vi "STA - Wave V5 Host_Wait_V2.2.vi"() -> ()   [LabVIEW 2015]
doc: "The continuous acquisition mode tells the FPGA to acquire points indefinitely until a stop command is issued or until an error is encountered (FIFO overflow, module underflow, and so on). \n\nIn this acquisition mode, explicitly call the appropriate rwfm_ConfigTiming VI and set the host application's data buffer to be many times larger than the read size. The examples use a 10X size by default. If the host application's data buffer fills, then the FPGA experiences a FIFO overflow causing the acquisition to stop."
uses:
  <vilib>/LabVIEW Targets/FPGA/cRIO/shared/nicrio_ModuleControls/nicrio_cRIO-9234_ConfigModeRing.ctl
  <vilib>/Platform/TimedLoop/XDataNode/timing_clust.ctl
  <vilib>/Platform/TimedLoop/XDataNode/nitl_modes.ctl
  <vilib>/Platform/TimedLoop/XDataNode/wakeup.ctl
  <vilib>/FPGAPlugInAG/cRIO-9112/niLvFpga_Open_cRIO-9112.vi
  <vilib>/rvi/interface/common/dynamic/niFpgaDynamicAddResources.vi
  <vilib>/Utility/error.llb/Error Cluster From Error Code.vi
  <vilib>/RVI Host/nirviSupport.llb/nirviErrorClusterFromErrorCode.vi
  <vilib>/rvi/errors/niLvFpgaAdjustHostInterfaceError.vi
  <vilib>/FPGAPlugInAG/Dynamic/niLvFpga_Close_Dynamic.vi
  <vilib>/rvi/interface/nirviOpenFPGA/nirviOpenFPGA.xnode
  FPGA Bitfiles/STA-WaveformV5_FPGATarget2_[FPGA]DeltaSigMa_sLRIAVfzKK0.lvbitx
  FPGA/[FPGA] DeltaSig Main V5.vi
  <vilib>/rvi/interface/nirviMethod/nirviMethod.xnode
  <vilib>/rvi/interface/nirviCloseFPGA/nirviCloseFPGA.xnode
  <vilib>/Platform/TimedLoop/XDataNode/XDataNode.xnode
  <vilib>/NI/cRIO Wfm/cRIO Wfm.lvlib
  <vilib>/rvi/interface/nirviMethod/StockFPGA_InlinedMethodWaitForSingleIRQ.vi
  <vilib>/FPGAPlugInAG/Dynamic/niLvFpga_WaitOnIrq_Dynamic.vi
  C:/Program Files (x86)/National Instruments/LabVIEW 2015/ProjectTemplates/Source/cRIOWfm/FPGA/[FPGA] SAR Acq Main.vi
  D/Documents/LabVIEW Data/STA - Waveform V0/FPGA Bitfiles/SARAcqMain_9074.lvbitx
  <vilib>/Platform/TimedLoop/XDataNode/XDNodeRunTimeDep.lvlib
panel:
  out "x > y?":bool
  out "error TDMS":errorcluster
  in  "base path":path=path "u:/"
  out "file path":path
  out "Size Waveform":i32
  out "size(s) 2":i32[](array[numeric])
  out "Y":sgl[][](array[numeric])
  in  "appended array 2":sgl[](array[numeric])
  out "appended array":sgl[](array[numeric])
  out "size(s)":i32[](array[numeric])
  out "i RT FIFO Read":i32
  out "Element 2":u32
  out "Element 1":u32
  out "transposed array":sgl[][](array[numeric])
  out "error out 2":errorcluster
  out "error out":errorcluster
  out "error fifo out":errorcluster
  out "Waveform Graph 2":sgl[][](graph)
  in  "Array":waveform(sgl)[](array[waveform])
  out "Waveform Graph":waveform(sgl)[](graph)
  out "Buffer Backlog":dbl caption="RT Buffer Backlog [%]" format="%#.2g"
  in  "Stop":bool
  in  "Amplitude":dbl(slide)=5.0 scale=0.0..10.0
  out "Time Measure":dbl
  out "data rate (S/s)":u32
  out "Channel Config":T2(array[cluster]) {"Input Configuration" items=["AC Coupled", "DC Coupled", "IEPE AC Coupled"]}
  in  "Samples per Read":i32=900
  # "Sampling Info"
  # "Channel Info"
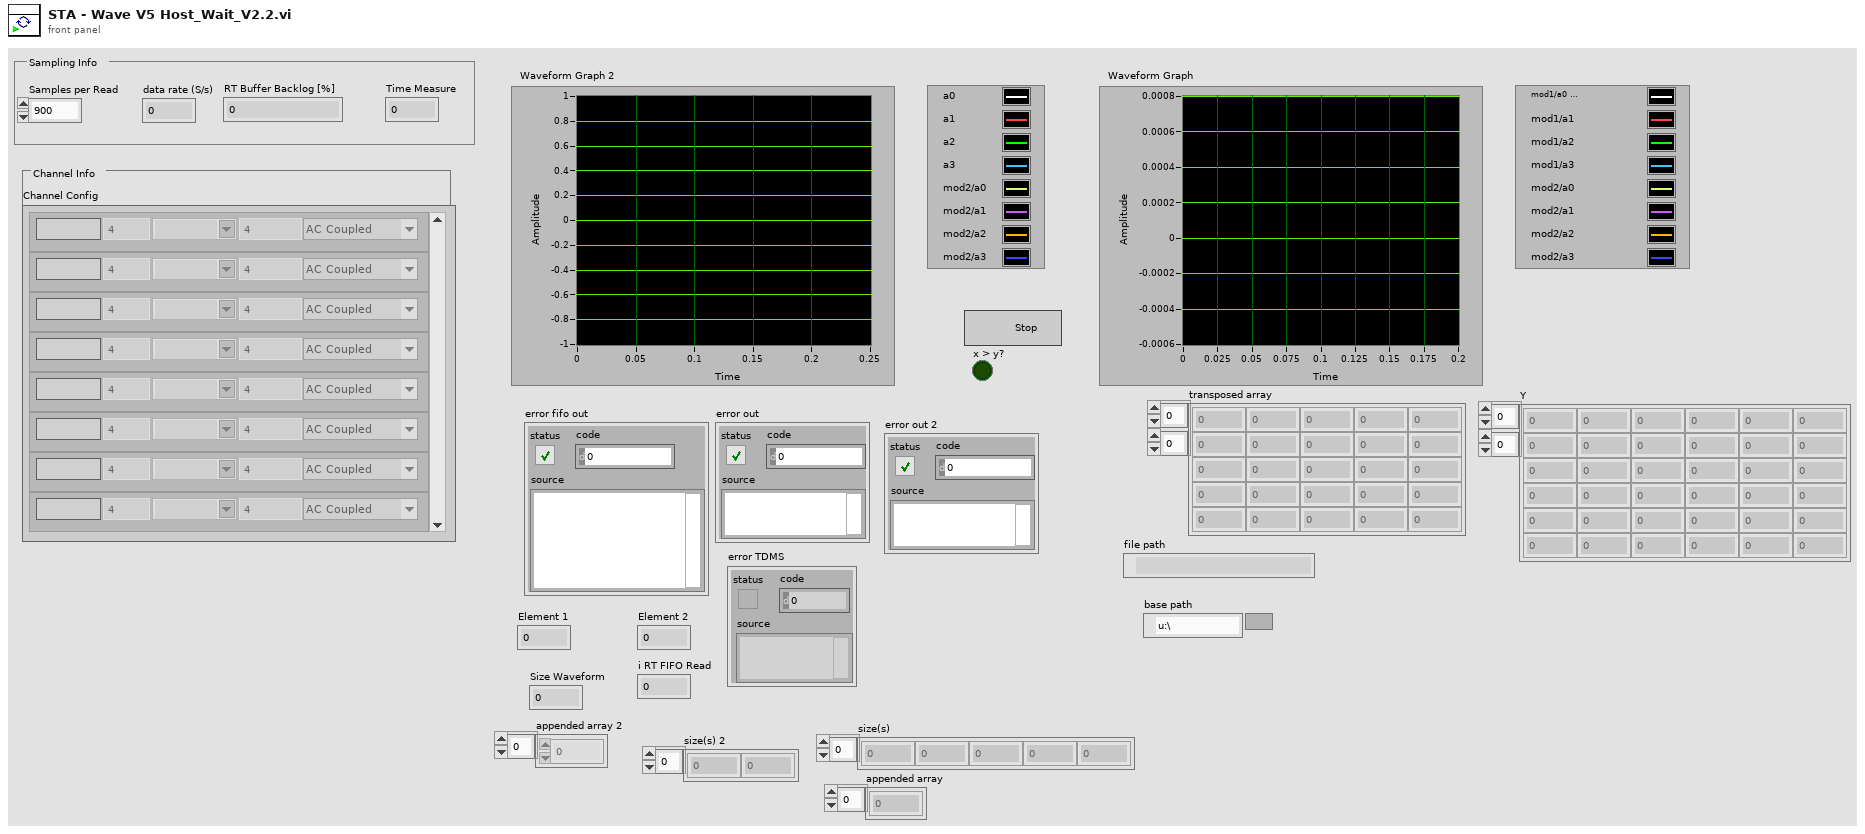
[diagram p1: front panel]
types:
  T1 = typedef "nicrio_cRIO-9234_ConfigModeRing.ctl" = u8
  T2 = cluster{"Channel Name":string, "Sensitivity mV_EU":dbl, "EU":string, "Input Configuration":T1, "dB Ref EU":dbl}[]
  T3 = enum16{"open", "open or create", "create or replace", "create", "open (read-only)"}
  T4 = typedef "XDNodeRunTimeDep.lvlib/timing_clust.ctl" = cluster{"Expected End [f-1]":u64, "Actual End [f-1]":u64, "Finished Late? [f-1]":bool, "Expected End [i-1]":u64, "Actual End [i-1]":u64, "Finished Late? [i-1]":bool, "Expected Start [i]":u64, "Actual Start [i]":u64, "Expected Start [f]":u64, "Actual Start [f]":u64, "Source Name":string, "Structure Name":string, "Period":i64, "Deadline":i64, "Offset":i64, "Start":i64, "Priority":i32, "Timeout":i32, "Mode":T5, "Wakeup Reason":T6, "Error":errorcluster, "Source Type":string, "Secondary Source Type":string, "Global End Time":u64, "Global Start Time":u64, "Frame Duration":u64, "Iteration Duration":u64, "Assigned CPU":i32, "I/O Scan Engine Mode":u32}
  T5 = typedef "XDNodeRunTimeDep.lvlib/nitl_modes.ctl" = enum32{"No Change", "Process missed periods, maintain original phase", "Discard missed periods, maintain original phase", "Process missed periods, ignore original phase", "Discard missed periods, ignore original phase"}
  T6 = typedef "XDNodeRunTimeDep.lvlib/wakeup.ctl" = enum32{"Normal", "Aborted", "Asynchronous wakeup", "Timing source error", "Timed loop error", "Timeout"}
  T7 = typedef "Acquisition and Logging Configuration_Waveform.ctl" = cluster{"Samples per Read":i32, "Number of Reads to Save":i32, "Data File Name":string, "TDMS Properties":T8[], "Number of Channels":i32, "Trigger - RMS Value":dbl, "Trigger - Channel":i32, "Trigger - Time (Minute)":i32, "Channel Config":cluster{"Channel Name":string, "Sensitivity mV_EU":dbl, "EU":string, "Input Configuration":T1, "dB Ref EU":dbl}[], "data rate (S/s)":u32, "Time Measure":dbl}
  T8 = typedef "TDMS Properties.ctl" = cluster{"Name":string, "Value":string}
  T9 = typedef "cRIO Wfm.lvlib/SamplingInfo.ctl" = cluster{"Number of Channels":i32, "Actual Samp Rate":dbl, "Chan Name Array":string[], "EU Chan Array":string[], "dB Ref Chan Array":dbl[]}
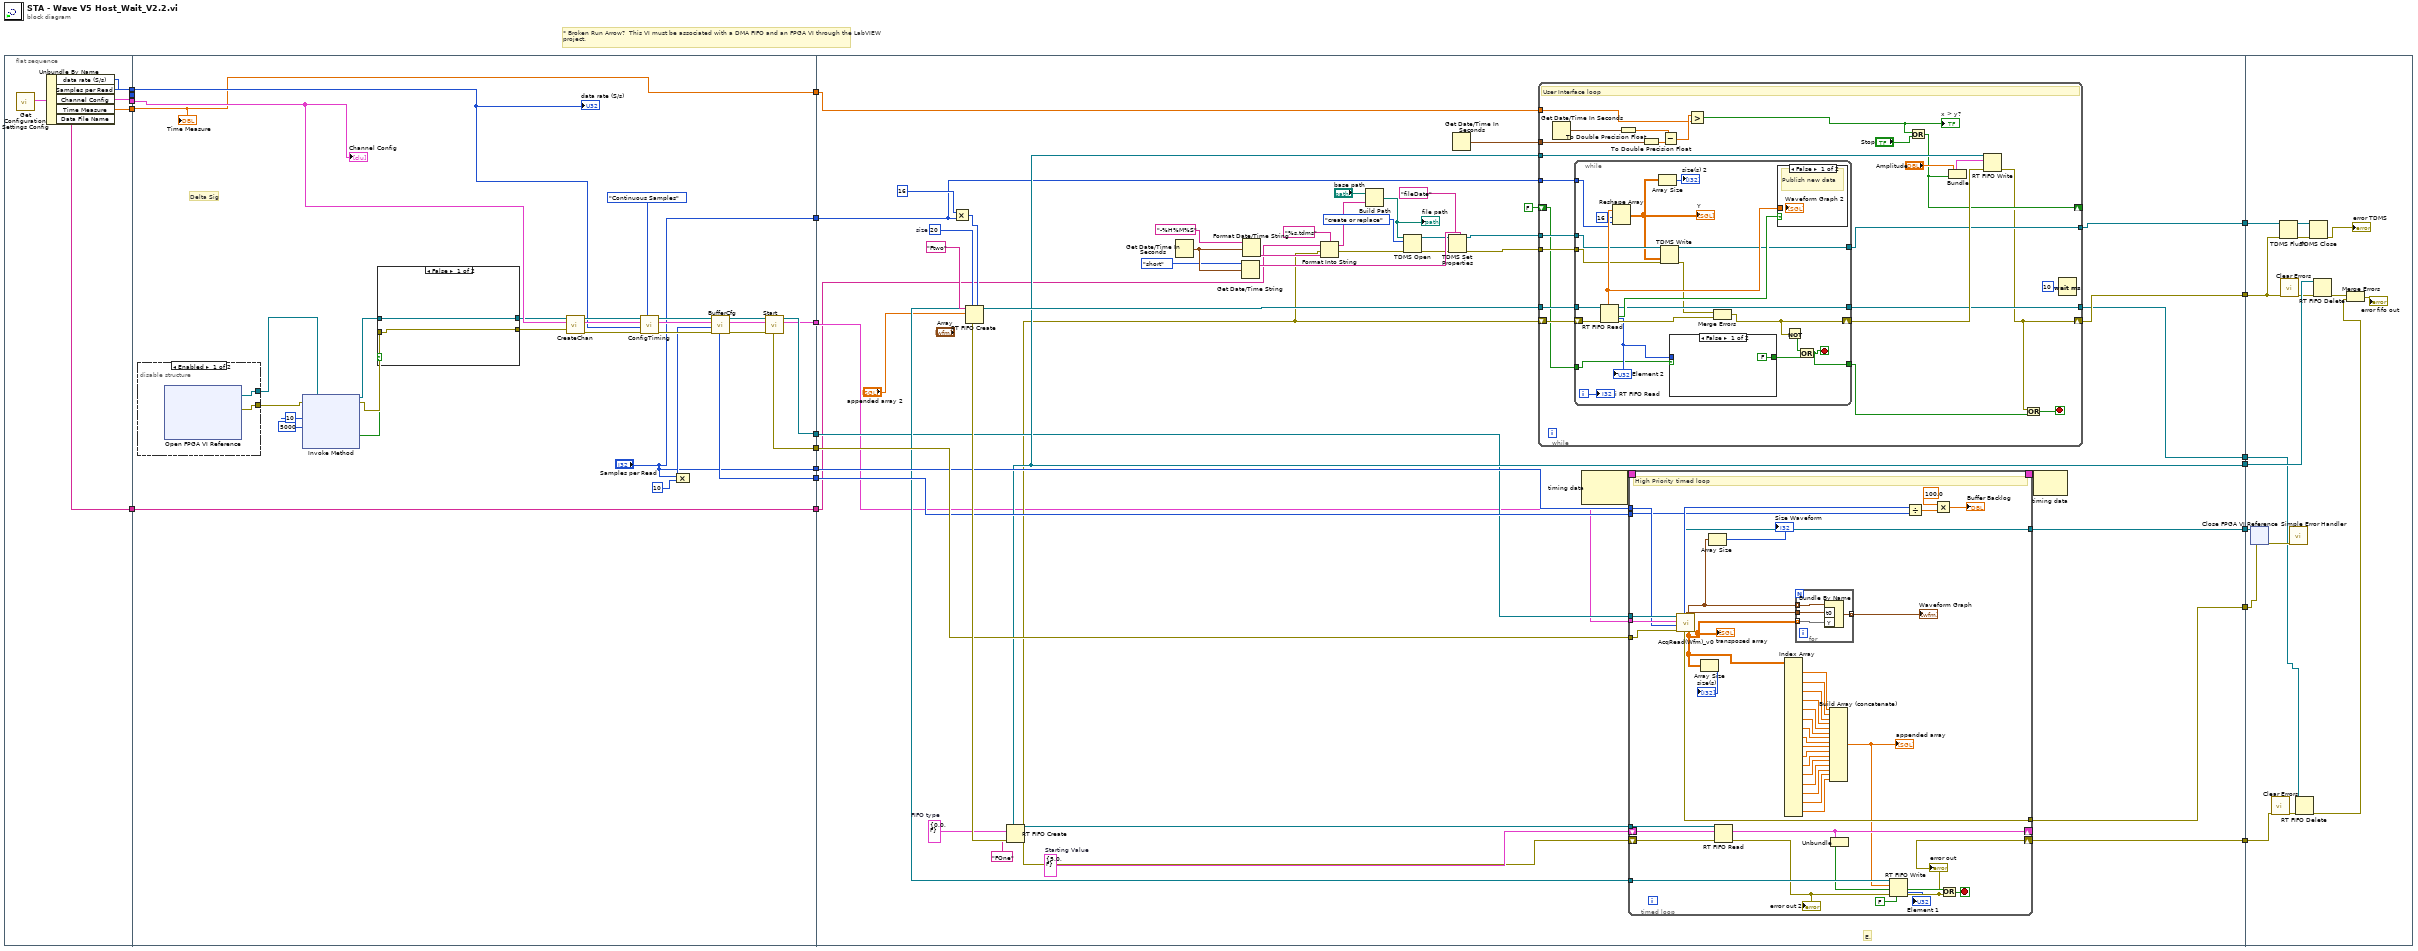
[diagram p0: block diagram]
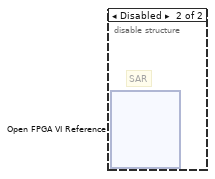
[diagram p2: hidden frame]
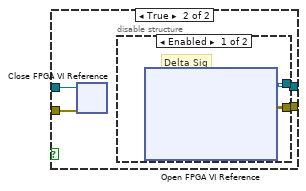
[diagram p3: hidden frame]
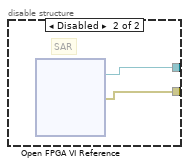
[diagram p4: hidden frame]
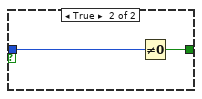
[diagram p5: hidden frame]
diagram:
  # "* Broken Run Arrow?  This VI must be associated with a DMA FIFO and an FPGA VI through the LabVIEW project."
  n1 = flat-sequence {
    tunnel: [w25] -> w20
    tunnel: [w24] -> w19
    tunnel: [w23] -> w18
    tunnel: [w22] -> w17
    tunnel: [w21] -> w10
    tunnel: w20 -> [w38]
    tunnel: w19 -> [_]
    tunnel: w18 -> [w37]
    tunnel: w17 -> [w31]
    tunnel: ["Samples per Read"] -> w16
    tunnel: [w31] -> w15
    tunnel: [w34] -> w14
    tunnel: [w33] -> w13
    tunnel: [w32] -> w12
    tunnel: [w30] -> w11
    tunnel: w10 -> [w29]
    tunnel: [w29] -> w9
    tunnel: ["Samples per Read"] -> w1
    tunnel: w16 -> [w109]
    tunnel: w15 -> [w73]
    tunnel: w14 -> [w99]
    tunnel: w13 -> [w77]
    tunnel: w12 -> [w110]
    tunnel: w11 -> [w108]
    tunnel: w9 -> [w76]
    tunnel: [w106] -> w8
    tunnel: [w105] -> w7
    tunnel: [w104] -> w6
    tunnel: [w100] -> w5
    tunnel: [w102] -> w4
    tunnel: [w101] -> w3
    tunnel: [w75] -> w2
    tunnel: w1 -> [w72]
    tunnel: w8 -> [w230]
    tunnel: w7 -> [w229]
    tunnel: w6 -> [w228]
    tunnel: w5 -> [w226]
    tunnel: w4 -> [w227]
    tunnel: w3 -> [w220]
    tunnel: w2 -> [w219]
    frame #0 {
      n2 = call "Get Configuration Settings Config.vi"() -> ("Configuration"=w26:T7)  [unwired: 10 in, 1 out]
      n3 = Unbundle By Name(w26) -> ("data rate (S/s)"=w25:u32, "Samples per Read"=w24:i32, "Channel Config"=w23:T2, "Time Measure"=w22:dbl, "Data File Name"=w21:string)
    }
    frame #1 {
      # "Delta Sig"
      n4 = disable-structure shown="Enabled" {
        disable-tunnel: [w58 _] -> w36
        disable-tunnel: [w57 _] -> w35
        frame Enabled {
          n5 = xnode "Open FPGA VI Reference"() -> ("FPGA VI Reference Out"=w58:refnum<k20>, "error out"=w57:errorcluster)  [unwired: 2 in]
        }
        frame Disabled {
          # "SAR"
          n6 = xnode "Open FPGA VI Reference"() -> ("FPGA VI Reference Out"=w60:refnum<k20>, "error out"=w59:errorcluster)  [unwired: 2 in]
        }
      }
      n7 = xnode "Invoke Method"("FPGA VI Reference In"=w36, "error in"=w35, "IRQ Number(s)"=10, "Timeout (ms)"=5000) -> ("FPGA VI Reference Out"=w54:refnum<k20>, "error out"=w55:errorcluster, "Timed Out"=w53:bool)  [unwired: 1 out]
      n8 = case shown="False" w53 {
        tunnel: w54 -> [w62 w66]
        tunnel: w55 -> [w61 w65]
        tunnel: [w62 w64] -> w28
        tunnel: [w61 w63] -> w56
        frame False {
        }
        frame True {
          n9 = xnode "Close FPGA VI Reference"("FPGA VI Reference In"=w66, "error in"=w65) -> ()  [unwired: 1 out]
          n10 = disable-structure shown="Enabled" {
            disable-tunnel: [w68 w70] -> w64
            disable-tunnel: [w67 w69] -> w63
            frame Enabled {
              # "Delta Sig"
              n11 = xnode "Open FPGA VI Reference"() -> ("FPGA VI Reference Out"=w68:refnum<k20>, "error out"=w67:errorcluster)  [unwired: 2 in]
            }
            frame Disabled {
              # "SAR"
              n12 = xnode "Open FPGA VI Reference"() -> ("FPGA VI Reference Out"=w70:refnum<k20>, "error out"=w69:errorcluster)  [unwired: 2 in]
            }
          }
        }
      }
      n13 = call <vilib>:"CreateChan.vi"("Dynamic FPGA Ref"=w28, "Channel Config"=w37, "error in"=w56) -> ("Dynamic FPGA Ref Out"=w44:refnum<k20>, "Sampling Info"=w45:T9, "error out"=w49:errorcluster)  [unwired: 5 in]
      n14 = call <vilib>:"ConfigTiming.vi"("Sample Mode"=enum16{"Finite Samples", "Continuous Samples"}."Continuous Samples", "error in"=w49, "Sample Rate"=w38, "Sampling Info In"=w45, "Dynamic FPGA Ref"=w44) -> ("error out"=w48:errorcluster, "Sampling Info Out"=w47:T9, "Dynamic FPGA Ref Out"=w46:refnum<k20>)  [unwired: 3 in, 1 out]
      n15 = Compound Arithmetic op=MULTIPLY("Samples per Read", 10 ("value")) -> (w42:i32)
      n16 = call <vilib>:"BufferCfg.vi"("error in"=w48, "Buffer Size [Samps per Chan]"=w42, "Sampling Info In"=w47, "Dynamic FPGA Ref"=w46) -> ("error out"=w41:errorcluster, "Buffer Size [Total Samples]"=w30:u32, "Sampling Info Out"=w43:T9, "Dynamic FPGA Ref Out"=w40:refnum<k20>)  [unwired: 4 out]
      n17 = call <vilib>:"Start.vi"("error in"=w41, "Sampling Info In"=w43, "Dynamic FPGA Ref"=w40) -> ("error out"=w32:errorcluster, "Sampling Info Out"=w33:T9, "Dynamic FPGA Ref Out"=w34:refnum<k20>)  [unwired: 6 out]
      "Channel Config" <- w37
      "data rate (S/s)" <- w38
      "Time Measure" <- w31
    }
    frame #2 {
      w111 = cluster{dbl, bool} {5.0, FALSE}  # Starting Value
      w112 = cluster{dbl, bool} {0.0, FALSE}  # FIFO type
      w113 = u32 20  # size
      # "E."
      n18 = Multiply(x=16 ("dimension size"), y=w72) -> (x*y=w96:i32)
      n19 = RT FIFO Create(0:"Ftwo" ("name (unnamed)"), 1:"appended array 2", 4:w113, 6:w96) -> (8:w103:refnum<k33>, 11:w114:errorcluster)  [unwired: 2 in, 3 out]
      n20 = RT FIFO Create(0:"FOne" ("name (unnamed)"), 1:w112, 3:w114) -> (8:w102:refnum<k33>, 11:w78:errorcluster)  [unwired: 2 in, 4 out]
      n21 = Get Date/Time In Seconds() -> (seconds since 1Jan1904=w93:timestamp)
      n22 = Get Date/Time String(date format (0)=enum16{"short", "long", "abbreviated"}."short", seconds (now)=w93) -> (date string=w94:string)  [unwired: 1 in, 1 out]
      n23 = Format Date/Time String(time format string (%c)="-%H%M%S", seconds (now)=w93) -> (date/time string=w86:string)  [unwired: 1 in]
      n24 = Format Into String(format string="%s.tdms", initial string=w76, error in=w78, w86) -> (resulting string=w83:string, error out=w92:errorcluster)
      n25 = Build Path(base path="base path", name or relative path=w83) -> (appended path=w89:path)
      "file path" <- w89
      n26 = TDMS Open(8:w92, 10:T3."create or replace" ("operation (0:open)"), 11:w89) -> (0:w87:errorcluster, 3:w88:refnum<k34>)  [unwired: 4 in]
      n27 = TDMS Set Properties(5:w94, 7:"fileDate" ("property names"), 8:w87, 11:w88) -> (0:w79:errorcluster, 3:w80:refnum<k34>)  [unwired: 2 in, 2 out]
      n28 = Get Date/Time In Seconds() -> (seconds since 1Jan1904=w74:timestamp)
      n29 = while "User Interface loop" {
        shift-right: [w171] -> w101
        shift-left: w78 -> [w192]
        tunnel: w102 -> [w191]
        tunnel: w103 -> [w193]
        tunnel: [w186] -> w100
        tunnel: w80 -> [w185]
        tunnel: w79 -> [w184]
        tunnel: [w183] -> w75
        tunnel: w74 -> [w182]
        tunnel: w73 -> [w177]
        tunnel: w72 -> [w174]
        shift-right: [w173] -> _
        shift-left: FALSE -> [w172]
        stop <- w169 stop-if-true
        # "User Interface loop"
        n30 = Get Date/Time In Seconds() -> (seconds since 1Jan1904=w181:timestamp)
        n31 = while {
          tunnel: w193 -> [w214]
          shift-right: [w201] -> w190
          shift-left: w192 -> [w213]
          tunnel: [w211] -> w186
          tunnel: w185 -> [w206]
          tunnel: w184 -> [w205]
          tunnel: [w200] -> w183
          tunnel: w174 -> [w199]
          tunnel: w172 -> [w196]
          tunnel: [w194] -> w170
          i -> [w210]
          stop <- w194 stop-if-true
          n32 = RT FIFO Read(0:w214, 3:w213) -> (7:w198:u32, 8:w211:refnum<k33>, 9:w209:sgl[], 10:w212:bool, 11:w202:errorcluster)  [unwired: 1 in, 1 out]
          "Element 2" <- w198
          n33 = Reshape Array(w209, 16 ("dimension size"), w199) -> (w204:sgl[][])
          "Y" <- w204
          n34 = Array Size(array=w204) -> (size(s)=→"size(s) 2":i32[])
          n35 = TDMS Write(0:w206, 9:w204, 11:w205) -> (4:w200:refnum<k34>, 15:w203:errorcluster)  [unwired: 3 in, 2 out]
          n36 = case shown="False" w196 {
            tunnel: w198 -> [_ w217]
            tunnel: [FALSE w216] -> w195
            frame False {
            }
            frame True {
              n37 = Not Equal To 0?(x=w217) -> (x != 0?=w216:bool)
            }
          }
          n38 = Merge Errors(w203, w202) -> (w201:errorcluster)
          n39 = case shown="False" w212 {
            tunnel: w209 -> [_ _]
            frame False {
              # "Publish new data"
            }
            frame True {
              # "No new data"
            }
          }
          n40 = Not(x=w201) -> (.not. x?=w197:bool)
          n41 = Or(x=w197, y=w195) -> (x .or. y?=w194:bool)
          "i RT FIFO Read" <- w210
        }
        n42 = To Double Precision Float(number=w181) -> (double precision float=w180:dbl)
        n43 = To Double Precision Float(number=w182) -> (double precision float=w179:dbl)
        n44 = Subtract(x=w180, y=w179) -> (x-y=w178:dbl)
        n45 = Greater?(x=w178, y=w177) -> (0:w176:bool)
        "x > y?" <- w176
        n46 = Or(x=w176, y="Stop") -> (x .or. y?=w173:bool)
        n47 = Bundle("Amplitude"="Amplitude", w173) -> (w187:cluster{"Amplitude":dbl, bool})  [unwired: 1 in]
        n48 = RT FIFO Write(0:w191, 1:w187, 3:w190) -> (11:w171:errorcluster)  [unwired: 2 in, 3 out]
        n49 = Or(x=w171, y=w170) -> (x .or. y?=w169:bool)
        n50 = Wait (ms)(milliseconds to wait=u32 10 ("millisecond multiple")) -> ()  [unwired: 1 out]
      }
      n51 = node-c288() -> (w116:T4)  [unwired: 1 in, 1 out]
      n52 = timed-loop "High Priority timed loop" {
        shift-left: w111 -> [w160]
        shift-right: [w156] -> _
        shift-right: [w140] -> w104
        shift-left: w78 -> [w157]
        timing: w116 -> [_]
        timing-out: [_] -> w115
        tunnel: w102 -> [w161]
        tunnel: w103 -> [w159]
        tunnel: w77 -> [w148]
        tunnel: w99 -> [w147]
        tunnel: w110 -> [w146]
        tunnel: w109 -> [w145]
        tunnel: w108 -> [w144]
        tunnel: [w142] -> w106
        tunnel: [w141] -> w105
        stop <- w154 stop-if-true
        # "High Priority timed loop"
        n53 = call <vilib>:"AcqRead(Wfm)_v0.vi"("error in"=w146, "Samps Read per Chan"=w145, "Sampling Info"=w148, "Dynamic FPGA Ref"=w147) -> ("error out"=w141:errorcluster, "Samples Remaining"=w153:u32, "time stamp"=w149:timestamp, "Dynamic FPGA Ref Out"=w142:refnum<k20>, "transposed array"=w136:sgl[][], "Array"=w118:waveform(sgl)[])  [unwired: 2 in]
        "transposed array" <- w136
        n54 = Array Size(array=w136) -> (size(s)=→"size(s)":i32[])
        n55 = Array Size(array=w118) -> (size(s)=→"Size Waveform":i32)
        n56 = RT FIFO Read(0:w161, 1:w160, 3:w157) -> (9:w156:cluster{dbl, bool}, 11:w158:errorcluster)  [unwired: 4 out]
        "error out 2" <- w158
        n57 = Index Array(array=w136) -> (element #1=w135:sgl[], element #2=w134:sgl[], element #3=w133:sgl[], element #4=w132:sgl[], element #5=w131:sgl[], element #6=w130:sgl[], element #7=w129:sgl[], element #8=w128:sgl[], element #9=w127:sgl[], element #10=w126:sgl[], element #11=w125:sgl[], element #12=w124:sgl[], element #13=w123:sgl[], element #14=w122:sgl[], element #15=w121:sgl[], element #16=w120:sgl[])  [unwired: 32 in]
        n58 = for {
          tunnel: w118 -> [w165] mode=indexing
          tunnel: w149 -> [w164]
          tunnel: [w163] -> w143 mode=indexing
          tunnel: w136 -> [w162] mode=indexing
          n59 = Bundle By Name(cluster=w165, "t0"=w164, "Y"=w162) -> (w163:waveform(sgl))
        }
        "Waveform Graph" <- w143
        n60 = Build Array (concatenate)(w135, w134, w133, w132, w131, w130, w129, w128, w127, w126, w125, w124, w123, w122, w121, w120) -> (w119:sgl[])
        "appended array" <- w119
        n61 = Unbundle(w156) -> (w155:bool)  [unwired: 1 out]
        n62 = RT FIFO Write(0:w159, 1:w119, 3:w158, 5:FALSE ("overwrite on timeout (T)")) -> (7:→"Element 1":u32, 11:w140:errorcluster)  [unwired: 3 out]
        "error out" <- w140
        n63 = Divide(x=w153, y=w144) -> (x/y=w152:dbl)
        n64 = Multiply(x=100.0, y=w152) -> (x*y=→"Buffer Backlog":dbl)
        n65 = Or(x=w155, y=w140) -> (x .or. y?=w154:bool)
      }
      n66 = node-c288(w115) -> ()  [unwired: 1 out]
    }
    frame #3 {
      n67 = xnode "Close FPGA VI Reference"("FPGA VI Reference In"=w230, "error in"=w229) -> ("error out"=w234:errorcluster)
      n68 = call <vilib>:"Clear Errors.vi"("error in (no error)"=w228) -> ("error out"=w231:errorcluster)  [unwired: 5 in, 1 out]
      n69 = TDMS Flush(4:w220, 7:w219) -> (0:w221:errorcluster, 3:w223:refnum<k34>)
      n70 = call <vilib>:"Clear Errors.vi"("error in (no error)"=w220) -> ("error out"=w225:errorcluster)  [unwired: 5 in, 1 out]
      n71 = call <vilib>:"Simple Error Handler.vi"("error in (no error)"=w234) -> ()  [unwired: 1 in, 8 out]
      n72 = RT FIFO Delete(0:w226, 3:w231) -> (11:w224:errorcluster)  [unwired: 1 in]
      n73 = TDMS Close(8:w221, 11:w223) -> (0:→"error TDMS":errorcluster)  [unwired: 1 out]
      n74 = RT FIFO Delete(0:w227, 3:w225) -> (11:w232:errorcluster)  [unwired: 1 in]
      n75 = Merge Errors(w232, w224) -> (→"error fifo out":errorcluster)
    }
  }
